vi "Switch_Initialize.vi"(11 "Semiconductor Module Context":T1) -> (0 "error out":errorcluster)   [LabVIEW 2014]
uses:
  <vilib>/NI_TestStand_SemiconductorModule/NI_TestStand_Semiconductor_Module.lvlibp/PinMap/General/SemiconductorModuleContext.ctl
  <instrlib>/niSwitch/niSwitch.LLB/niSwitch Topologies.ctl
  <vilib>/NI_TestStand_SemiconductorModule/NI_TestStand_Semiconductor_Module.lvlibp
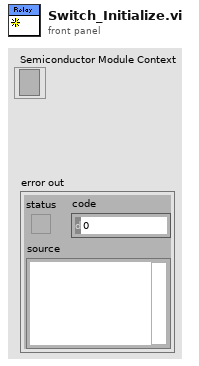
[diagram p1: front panel]
types:
  T1 = typedef "NI_TestStand_Semiconductor_Module.lvlibp/SemiconductorModuleContext.ctl" = refnum<k7>
  T2 = typedef "niSwitch Topologies.ctl" = string
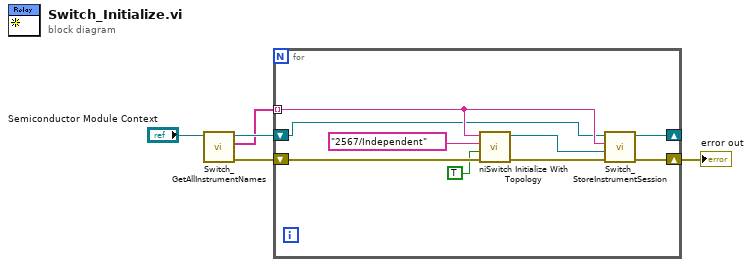
[diagram p0: block diagram]
diagram:
  n1 = call "Switch_GetAllInstrumentNames.vi"("Semiconductor Module Context"="Semiconductor Module Context") -> ("error out"=w3:errorcluster, "Instrument Names"=w1:string[], "Semiconductor Module Context Out"=w4:T1)  [unwired: 7 in, 1 out]
  n2 = for {
    shift-right: [w14] -> w2
    shift-left: w3 -> [w12]
    shift-right: [w13] -> _
    shift-left: w4 -> [w9]
    tunnel: w1 -> [w11] mode=indexing
    n3 = call <instrlib>:"niSwitch Initialize With Topology.vi"("error in (no error)"=w12, "reset device (boolean value)"=TRUE, "topology name"=T2 "2567/Independent", "resource name"=w11) -> ("error out"=w10:errorcluster, "instrument handle out"=w7:refnum<k15>)  [unwired: 6 in]
    n4 = call "Switch_StoreInstrumentSession.vi"("error in (no error)"=w10, "Instrument Session"=w7, "Instrument Name"=w11, "Semiconductor Module Context"=w9) -> ("error out"=w14:errorcluster, "Semiconductor Module Context Out"=w13:T1)  [unwired: 6 in]
  }
  "error out" <- w2
